vi "Rinocloud_HTTP_children.vi"(3 "error in (no error)":errorcluster, 4 "Pagination variables":cluster{"limit":dbl, "offset":dbl}={"limit"=15.0, "offset"=0.0}, 5 "id":string) -> (0 "error out":errorcluster, 1 "Status":T2={"headers"="", "body"="", "ID"="", "Saved"=TRUE}, 2 "metadata array":T1(array[cluster]))   [LabVIEW 2011, in "Rinocloud Library.lvlib"]
uses:
  Rinocloud Library.lvlib
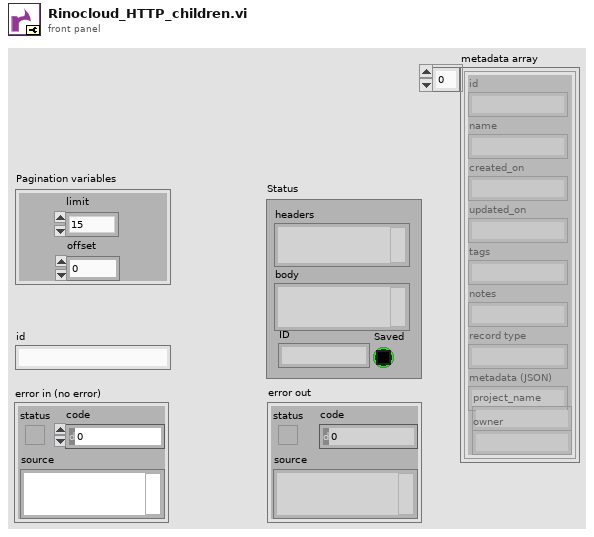
[diagram p1: front panel]
types:
  T1 = cluster{"id":string, "name":string, "created_on":string, "updated_on":string, "tags":string, "notes":string, "record type":string, "metadata (JSON)":string, "project_name":string, "owner":string}[]
  T2 = cluster{"headers":string, "body":string, "ID":string, "Saved":bool}
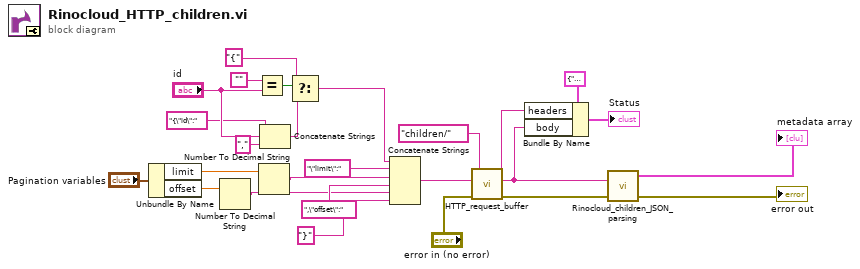
[diagram p0: block diagram]
diagram:
  n1 = Unbundle By Name("Pagination variables") -> ("limit"=w11:dbl, "offset"=w10:dbl)
  n2 = Number To Decimal String(number=w10) -> (decimal integer string=w1:string)  [unwired: 1 in]
  n3 = Equal?(x="", y="id") -> (x = y?=w23:bool)
  n4 = Number To Decimal String(number=w11) -> (decimal integer string=w2:string)  [unwired: 1 in]
  n5 = Concatenate Strings("{\"id\":" ("string"), "id", "," ("string")) -> (w24:string)
  n6 = Select(t="{", s=w23, f=w24) -> (s? t:f=w4:string)
  n7 = Concatenate Strings(w4, "\"limit\":" ("string"), w2, ",\"offset\":" ("string"), w1, "}" ("string")) -> (w3:string)
  n8 = call "HTTP_request_buffer.vi"("error in (no error)"="error in (no error)", "JSON payload"=w3, "Endpoint"="children/") -> ("error out"=w20:errorcluster, "body"=w21:string, "headers"=w19:string)  [unwired: 2 in]
  n9 = Bundle By Name(cluster=T2 {"headers"="", "body"="", "ID"="", "Saved"=TRUE} ("Status 2"), "headers"=w19, "body"=w21) -> (→"Status":T2)
  n10 = call "Rinocloud_children_JSON_parsing.vi"("error in (no error)"=w20, "JSON string"=w21) -> ("error out"=→"error out":errorcluster, "metadata array"=→"metadata array":T1)  [unwired: 2 in]
